vi "题目8.vi"() -> ()   [LabVIEW 2017]
panel:
  out "数值":dbl
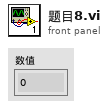
[diagram p1: front panel]
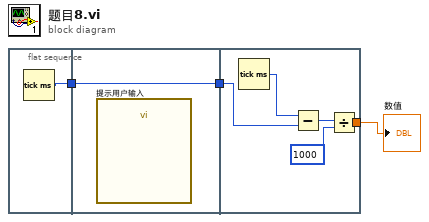
[diagram p0: block diagram]
diagram:
  n1 = flat-sequence {
    tunnel: [w4] -> w2
    tunnel: [w5] -> w3
    tunnel: w2 -> [w5]
    tunnel: w3 -> [w9]
    tunnel: [w6] -> w1
    frame #0 {
      n2 = Tick Count (ms)() -> (millisecond timer value=w4:u32)
    }
    frame #1 {
      n3 = call "提示用户输入"() -> ()  [unwired: 17 in, 3 out]
    }
    frame #2 {
      n4 = Tick Count (ms)() -> (millisecond timer value=w10:u32)
      n5 = Subtract(x=w10, y=w9) -> (x-y=w8:u32)
      n6 = Divide(x=w8, y=u32 1000) -> (x/y=w6:dbl)
    }
  }
  "数值" <- w1
